vi "EncoderRateToRPM.vi"(10 "Enum":enum16{"Through Bore", "Mag"}(ring), 11 "EncoderRate":dbl) -> (2 "RPM":dbl, 3 "RPS":dbl)   [LabVIEW 2019]
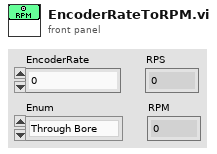
[diagram p1: front panel]
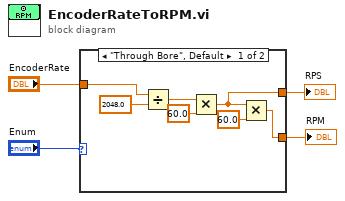
[diagram p0: block diagram]
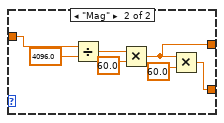
[diagram p2: hidden frame]
diagram:
  n1 = case shown="\"Through Bore\", Default" "Enum" {
    tunnel: "EncoderRate" -> [w7 w18]
    tunnel: [w6 w13] -> w2
    tunnel: [w5 w12] -> w1
    frame "Through Bore", Default {
      n2 = Divide(x=w7, y=2048.0) -> (x/y=w11:dbl)
      n3 = Multiply(x=w11, y=60.0) -> (x*y=w6:dbl)
      n4 = Multiply(x=w6, y=60.0) -> (x*y=w5:dbl)
    }
    frame "Mag" {
      n5 = Divide(x=w18, y=4096.0) -> (x/y=w14:dbl)
      n6 = Multiply(x=w14, y=60.0) -> (x*y=w13:dbl)
      n7 = Multiply(x=w13, y=60.0) -> (x*y=w12:dbl)
    }
  }
  "RPM" <- w1
  "RPS" <- w2
